vi "Main.vi"(8 "error in (no error)":errorcluster, 10 "UIEvents":refnum<user-event>) -> (0 "error out":errorcluster, 3 "ModuleQ Out":refnum<queue>)   [LabVIEW 2020, in "Controller.lvlib"]
doc: "Use this template to build a producer/consumer design pattern with events to produce queue items. Use this design pattern instead of the User Interface Event Handler pattern for user interfaces when you want to execute code asynchronously in response to an event without slowing the user interface responsiveness."
uses:
  Controller.lvlib
  Controls/ConsummerLoopData.ctl
  Controls/EventLoopData.ctl
  Controls/QMessage.ctl
  Support/UserEvents/Controls/EventMessage.ctl
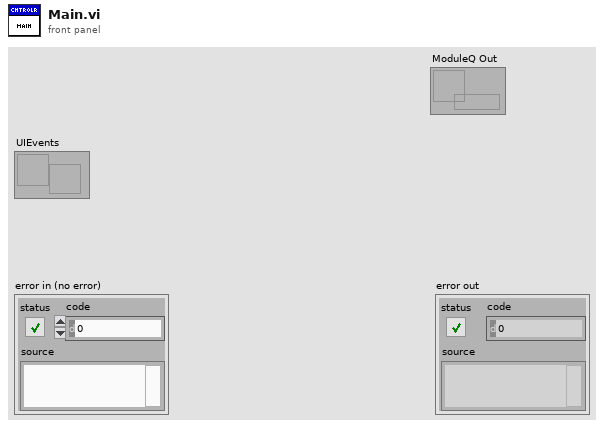
[diagram p1: front panel]
types:
  T1 = typedef "Controller.lvlib/QMessage.ctl" = cluster{"Message":string, "Data":variant}
  T2 = typedef "Controller.lvlib/EventLoopData.ctl" = cluster{"DummyData":dbl}
  T3 = typedef "Controller.lvlib/ConsummerLoopData.ctl" = cluster{"Error File Refnum":refnum<file>}
  T4 = typedef "EventMessage.ctl" = cluster{"Command":string, "Data":variant}
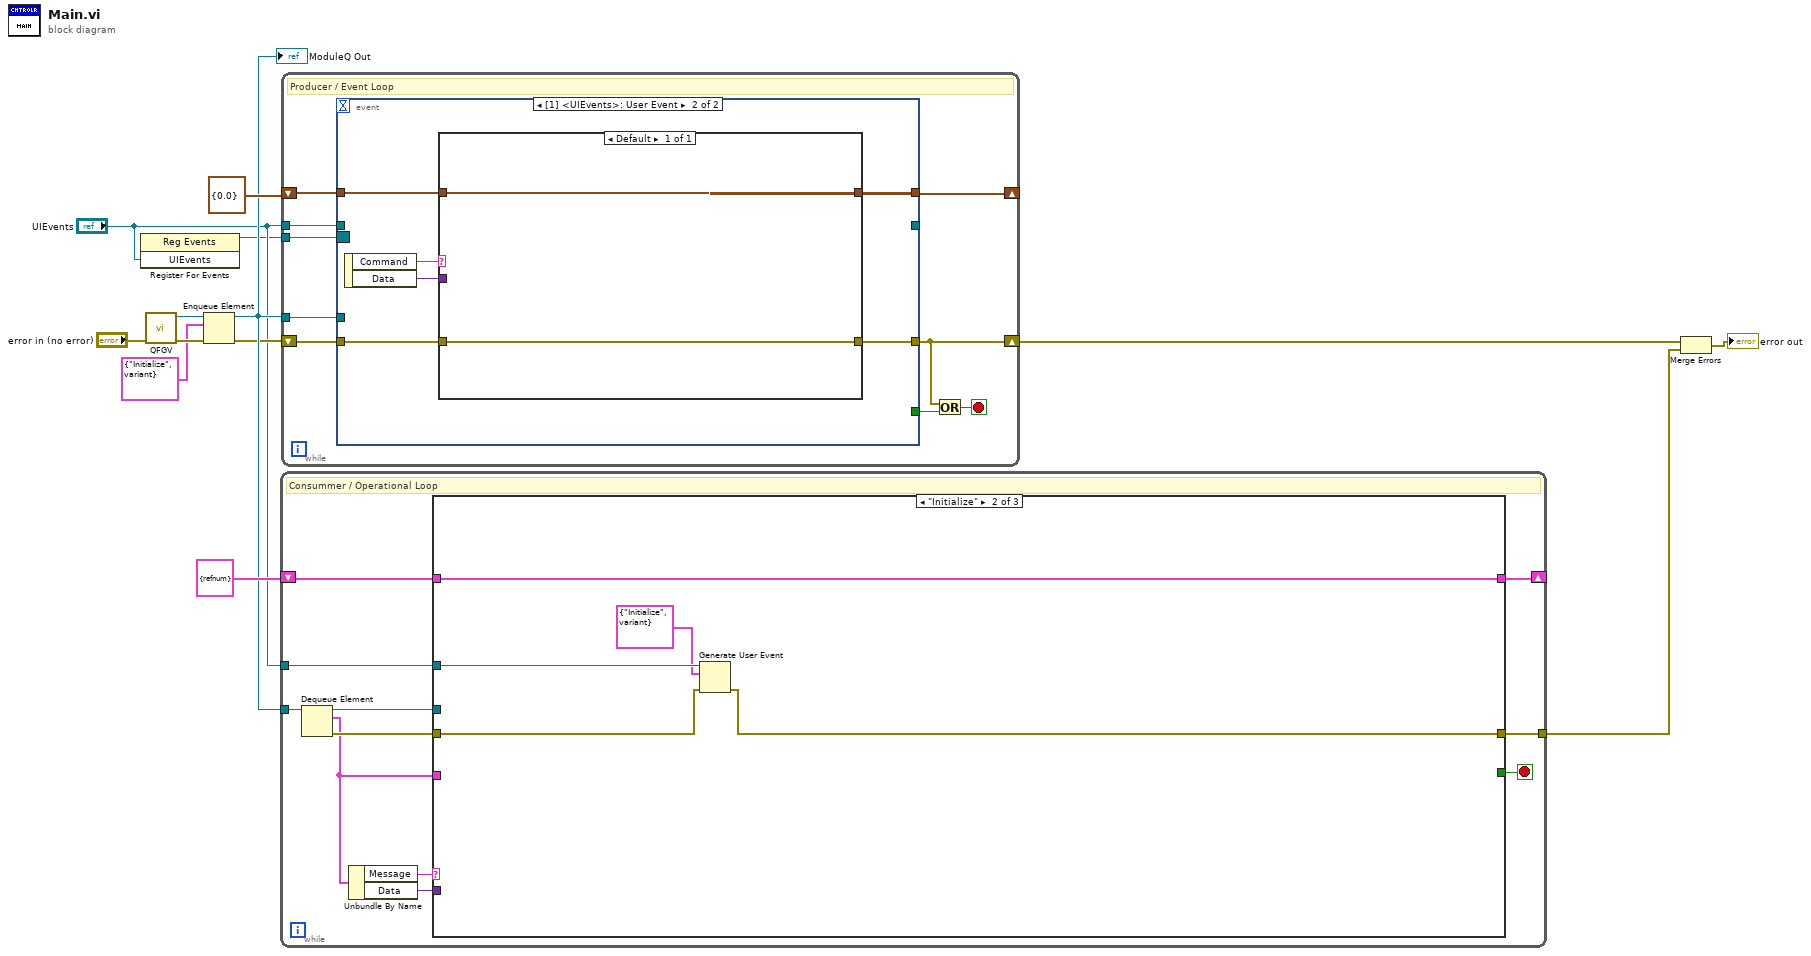
[diagram p0: block diagram]
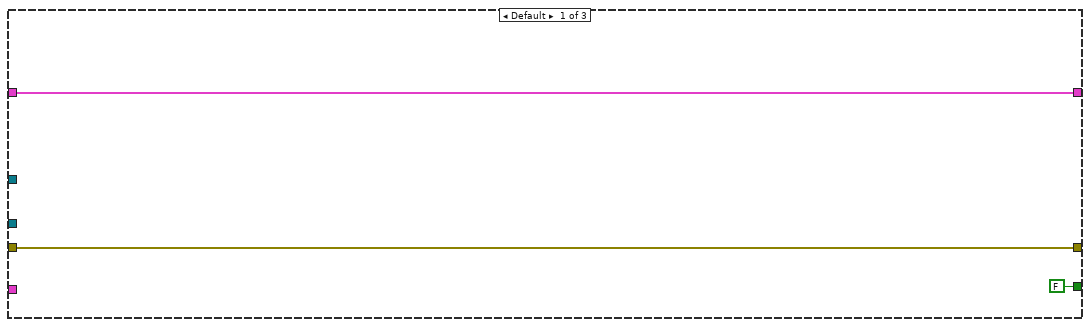
[diagram p2: hidden frame]
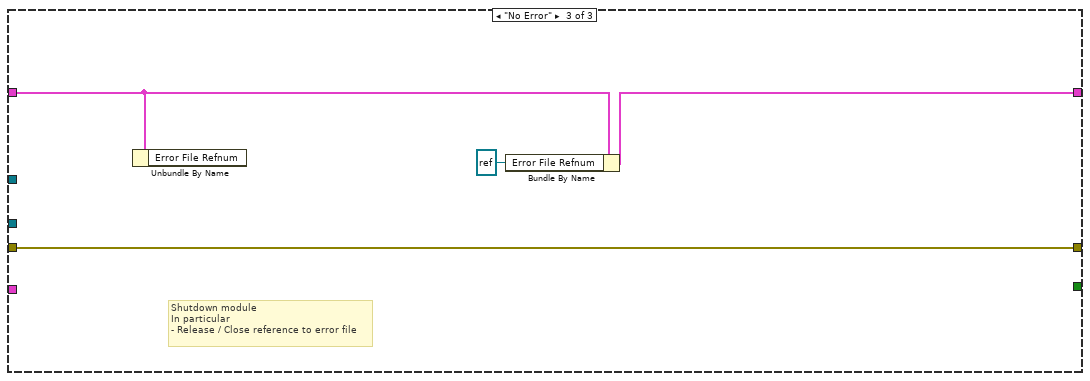
[diagram p3: hidden frame]
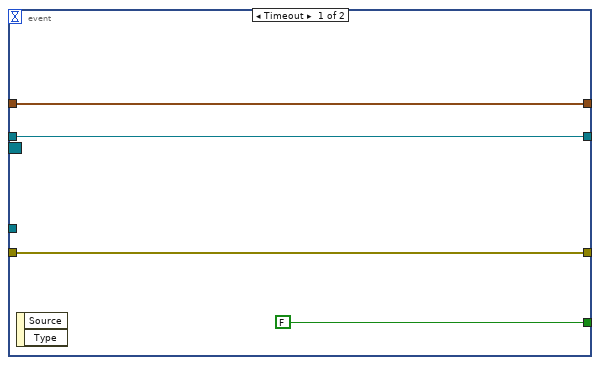
[diagram p4: hidden frame]
diagram:
  n1 = register-events("UIEvents") -> (reference out=w1:refnum<event-registration>)  [unwired: 2 in, 1 out]
  n2 = call "QFGV.vi"("error in (no error)"="error in (no error)") -> ("error out"=w7:errorcluster, "ModuleQ"=w6:refnum<queue>)  [unwired: 9 in]
  n3 = Enqueue Element(queue=w6, element=T1 {"Message"="Initialize", "Data"=variant}, error in (no error)=w7) -> (queue out=w5:refnum<queue>, error out=w4:errorcluster)  [unwired: 1 in, 1 out]
  "ModuleQ Out" <- w5
  n4 = while {
    tunnel: w5 -> [w24]
    shift-right: [w22] -> _
    shift-left: T3 {"Error File Refnum"=refnum} -> [w21]
    tunnel: [w19] -> w12
    tunnel: "UIEvents" -> [w14]
    stop <- w23 stop-if-true
    # "Consummer / Operational Loop"
    n5 = Dequeue Element(queue=w24) -> (queue out=w18:refnum<queue>, element=w17:T1, error out=w20:errorcluster)  [unwired: 2 in, 1 out]
    n6 = Unbundle By Name(w17) -> ("Message"=w16:string, "Data"=w15:variant)
    n7 = case shown="\"Initialize\"" w16 {
      tunnel: [FALSE _ _] -> w23
      tunnel: [w26 w32 w34] -> w22
      tunnel: w21 -> [w26 w32 w35]
      tunnel: w20 -> [w25 w29 w36]
      tunnel: [w25 w28 w36] -> w19
      tunnel: w18 -> [_ _ _]
      tunnel: w17 -> [_ _ _]
      tunnel: w15 -> [_ _ _]
      tunnel: w14 -> [_ w31 _]
      frame Default {
      }
      frame "Initialize" {
        n8 = Generate User Event(user event=w31, event data cluster=T4 {"Command"="Initialize", "Data"=variant} ("event data"), error in=w29) -> (error out=w28:errorcluster)  [unwired: 1 in, 1 out]
      }
      frame "No Error" {
        # "Shutdown module\nIn particular\n- Release / Close reference to error file"
        n9 = Unbundle By Name(w35) -> ()  [unwired: 1 out]
        n10 = Bundle By Name(cluster=w35, "Error File Refnum"=refnum<file> refnum) -> (w34:T3)
      }
    }
  }
  n11 = while {
    shift-right: [w41] -> w11
    shift-left: w4 -> [w44]
    tunnel: w5 -> [w45]
    shift-right: [w40] -> _
    shift-left: T2 {"DummyData"=0.0} -> [w39]
    tunnel: "UIEvents" -> [w38]
    tunnel: w1 -> [w37]
    stop <- w42 stop-if-true
    # "Producer / Event Loop"
    n12 = event shown="[1] <UIEvents>: User Event" {
      selector: w37 -> [_ _]
      dyn-events: _ -> [_ _]
      timeout: _ -> [_ _]
      tunnel: w45 -> [_ _]
      tunnel: w44 -> [w48 w50]
      tunnel: [w48 w51] -> w41
      tunnel: [FALSE ("stop") _] -> w43
      tunnel: [w49 w55] -> w40
      tunnel: w39 -> [w49 w54]
      tunnel: [w46 _] -> _
      tunnel: w38 -> [w46 _]
      event Timeout {
        n13 = event-data() -> ()  [unwired: 1 in, 2 out]
      }
      event User Event {
        n14 = event-data() -> ("Command"=w53:string, "Data"=w52:variant)  [unwired: 1 in]
        n15 = case shown="Default" w53 {
          tunnel: [w57] -> w55
          tunnel: w54 -> [w57]
          tunnel: w52 -> [_]
          tunnel: [w56] -> w51
          tunnel: w50 -> [w56]
          frame Default {
          }
        }
      }
    }
    n16 = Or(x=w41, y=w43) -> (x .or. y?=w42:bool)
  }
  n17 = Merge Errors(w11, w12) -> (→"error out":errorcluster)
